vi "main.vi"() -> ()   [LabVIEW 2021]
uses:
  data_cluster_typedef.ctl
  states_enum_typedef.ctl
  <vilib>/Utility/file.llb/Write Delimited Spreadsheet (DBL).vi
  <vilib>/Instr/_visa.llb/VISA Configure Serial Port (Instr).vi
  <vilib>/Utility/file.llb/Read Delimited Spreadsheet (DBL).vi
panel:
  out "XY Graph":cluster{"Time":dbl[], "Displacement":dbl[]}(graph)
  out "Connected?":bool
  in  "Serial Port":refnum<visa-resource-name>
  in  "Disconnect":bool
  in  "Connect":bool
  in  "Clear":bool
  in  "Save":bool
  in  "Load":bool
  in  "Exit":bool
  # "Creep Deformation"
  # "1) Connect your creep machine to the computer\n2) Select the appropriate serial port from the list\n3) Click \"Connect\"\n4) Run your experiment\n5) Save the data if desired, then clear the chart\n6) When all experiments are done, click \"Disconnect\""
  # "V1.1"
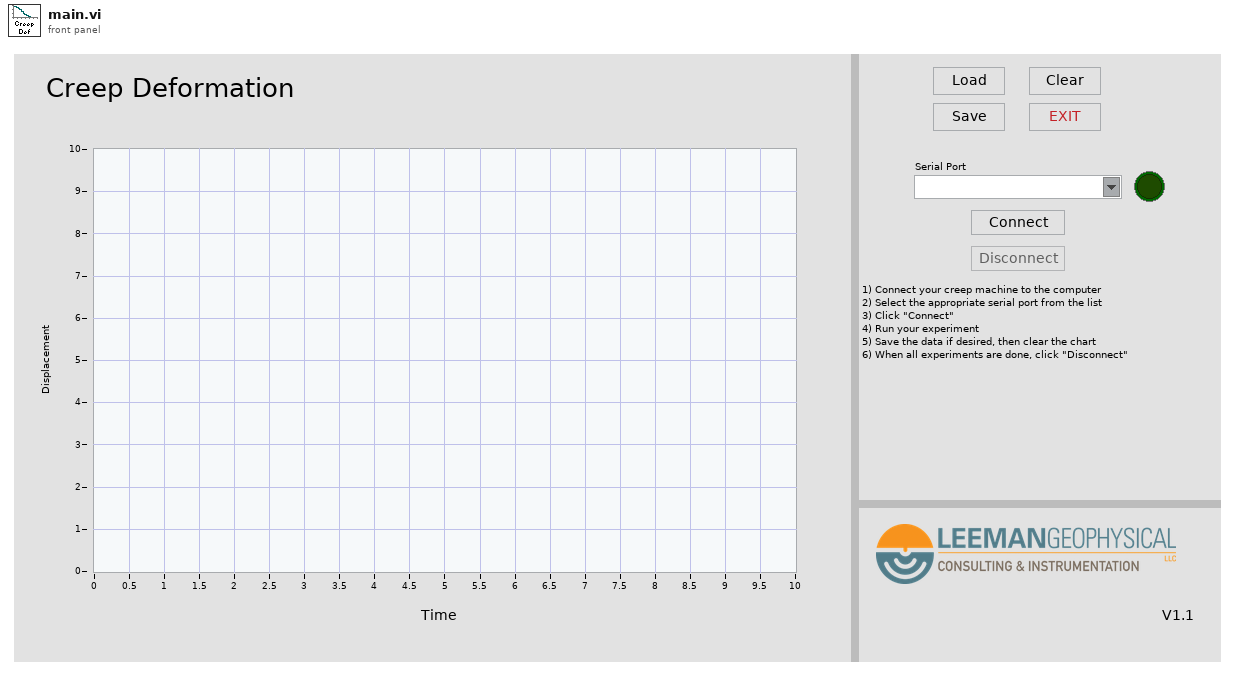
[diagram p1: front panel]
types:
  T1 = enum8{"Enabled", "Disabled", "Disabled and Grayed Out"}
  T2 = typedef "states_enum_typedef.ctl" = enum16{"Shutdown", "Update", "Initialize", "Clear", "Save", "Connect", "Disconnect", "Load", "Wait"}
  T3 = typedef "data_cluster_typedef.ctl" = cluster{"Time":dbl[], "Displacement":dbl[]}
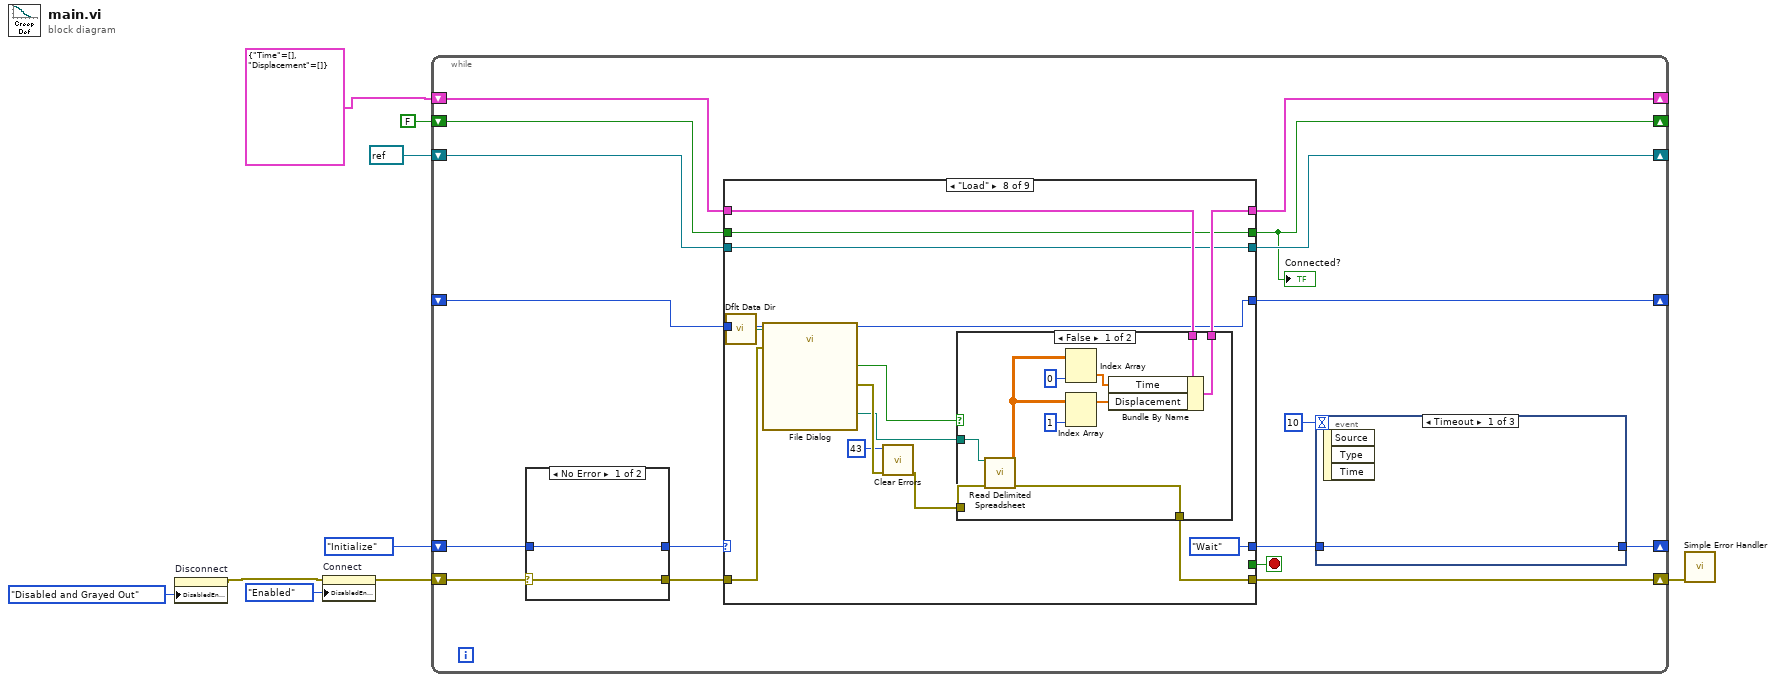
[diagram p0: block diagram]
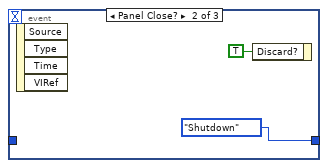
[diagram p2: hidden frame]
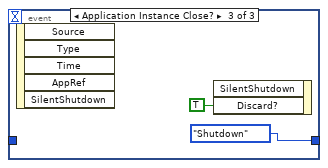
[diagram p3: hidden frame]
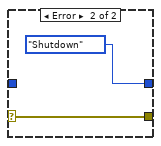
[diagram p4: hidden frame]
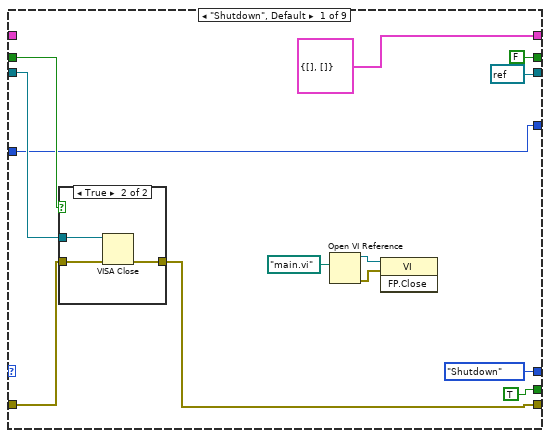
[diagram p5: hidden frame]
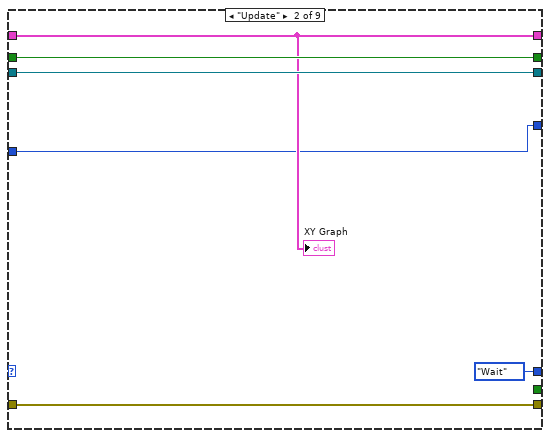
[diagram p7: hidden frame]
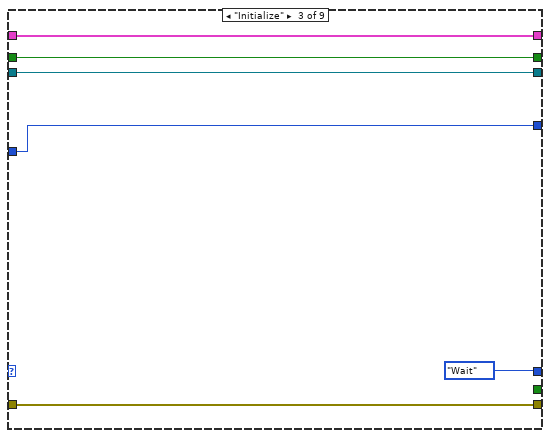
[diagram p8: hidden frame]
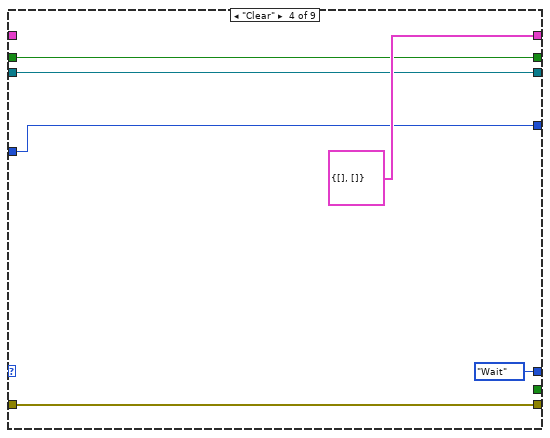
[diagram p9: hidden frame]
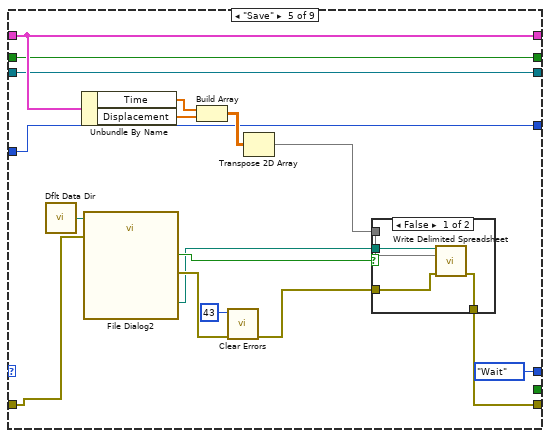
[diagram p10: hidden frame]
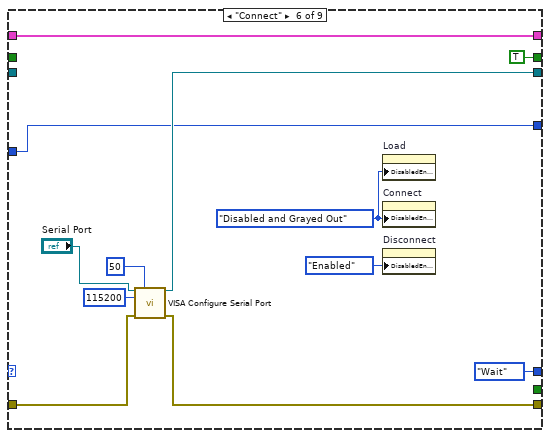
[diagram p12: hidden frame]
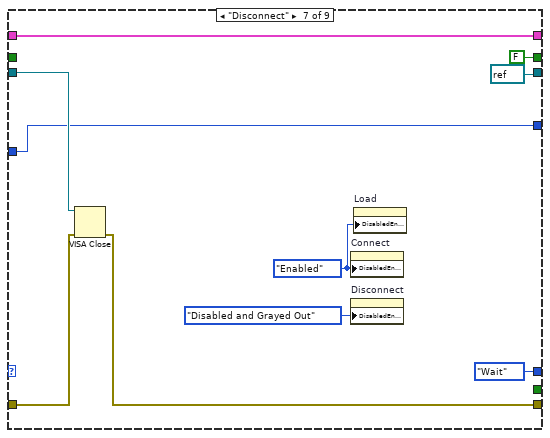
[diagram p13: hidden frame]
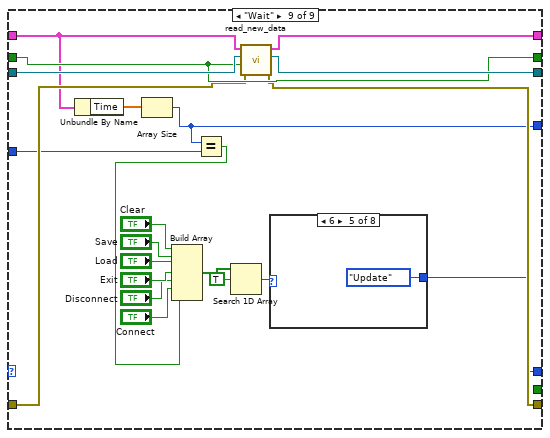
[diagram p15: hidden frame]
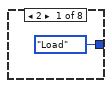
[diagram p16: hidden frame]
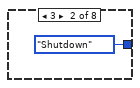
[diagram p17: hidden frame]
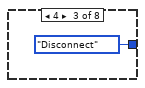
[diagram p18: hidden frame]
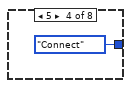
[diagram p19: hidden frame]
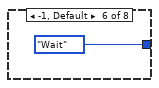
[diagram p20: hidden frame]
diagram:
  n1 = property on="Disconnect" class="Bool"("DisabledEnum"=T1."Disabled and Grayed Out" ("Disabled")) -> (error out=w2:errorcluster)  [unwired: 2 in, 1 out]
  n2 = property on="Connect" class="Bool"(error in=w2, "DisabledEnum"=T1."Enabled" ("Disabled")) -> (error out=w1:errorcluster)  [unwired: 1 in, 1 out]
  n3 = while {
    shift-right: [w11] -> _
    shift-left: states_enum_typedef."Initialize" -> [w25]
    shift-right: [w17] -> w5
    shift-left: w1 -> [w26]
    shift-right: [w19] -> _
    shift-left: T3 {"Time"=[], "Displacement"=[]} -> [w22]
    shift-right: [w16] -> _
    shift-left: FALSE -> [w21]
    shift-right: [w18] -> _
    shift-left: refnum<visa-resource-name> refnum ("Serial Port") -> [w20]
    shift-right: [w14] -> _
    shift-left: _ -> [w13]
    stop <- w15 stop-if-true
    n4 = case shown="No Error" w26 {
      selector: w26 -> [w32 w34]
      tunnel: w25 -> [w33 _]
      tunnel: [w33 states_enum_typedef."Shutdown"] -> w24
      tunnel: [w32 w34] -> w23
      frame No Error {
      }
      frame Error {
      }
    }
    n5 = case shown="\"Load\"" w24 {
      tunnel: w23 -> [w46 w55 w61 w66 w74 w101 w113 w118 w148]
      tunnel: w22 -> [_ w54 w64 _ w81 w98 w110 w128 w145]
      tunnel: w21 -> [w48 w58 w63 w69 w80 _ _ w126 w149]
      tunnel: w20 -> [w47 w57 w62 w68 w79 _ w114 w125 w150]
      tunnel: [T3 {"Time"=[], "Displacement"=[]} ("Data Cluster Out") w54 w64 T3 {"Time"=[], "Displacement"=[]} w81 w98 w110 w127 w152] -> w19
      tunnel: [FALSE w58 w63 w69 w80 TRUE FALSE w126 w149] -> w16
      tunnel: [refnum<visa-resource-name> refnum ("VISA out") w57 w62 w68 w79 w99 refnum<visa-resource-name> refnum ("VISA resource name out") w125 w151] -> w18
      tunnel: [w40 w55 w61 w66 w83 w100 w112 w124 w147] -> w17
      tunnel: [states_enum_typedef."Shutdown" states_enum_typedef."Wait" states_enum_typedef."Wait" states_enum_typedef."Wait" states_enum_typedef."Wait" states_enum_typedef."Wait" states_enum_typedef."Wait" states_enum_typedef."Wait" w146] -> w10
      tunnel: [TRUE _ _ _ _ _ _ _ _] -> w15
      tunnel: [w36 w53 w59 w65 w78 w94 w106 w122 w143] -> w14
      tunnel: w13 -> [w36 w53 w59 w65 w78 w94 w106 w122 w142]
      frame "Shutdown", Default {
        n6 = case shown="True" w48 {
          tunnel: w47 -> [_ w52]
          tunnel: w46 -> [w49 w51]
          tunnel: [w49 w50] -> w40
          frame False {
          }
          frame True {
            n7 = VISA Close(VISA resource name=w52, error in (no error)=w51) -> (error out=w50:errorcluster)
          }
        }
        n8 = Open VI Reference(vi path=path "main.vi") -> (vi reference=w38:refnum<vi>, error out=w37:errorcluster)  [unwired: 5 in]
        n9 = invoke class="VI" method="FP.Close"(reference=w38, error in=w37) -> ()  [unwired: 1 in, 3 out]
      }
      frame "Update" {
        "XY Graph" <- w54
      }
      frame "Initialize" {
      }
      frame "Clear" {
      }
      frame "Save" {
        n10 = call <vilib>:"Dflt Data Dir.vi"() -> ("App:Default Data Directory"=w77:path)
        n11 = Unbundle By Name(w81) -> ("Time"=w87:dbl[], "Displacement"=w86:dbl[])
        n12 = call "File Dialog2"("start path"=w77, "error in"=w74) -> ("selected path"=w71:path, "cancelled"=w73:bool, "error out"=w76:errorcluster)  [unwired: 10 in, 1 out]
        n13 = Build Array(w87, w86) -> (w85:dbl[][])
        n14 = call <vilib>:"Clear Errors.vi"("error in (no error)"=w76, "specific error code to clear (0: all)"=43) -> ("error out"=w72:errorcluster)  [unwired: 4 in, 1 out]
        n15 = Transpose 2D Array(2D array=w85) -> (transposed array=w84:dbl[][])
        n16 = case shown="False" w73 {
          tunnel: w84 -> [w91 _]
          tunnel: [w90 w92] -> w83
          tunnel: w72 -> [w89 w92]
          tunnel: w71 -> [w88 _]
          frame False {
            n17 = call-poly <vilib>:"Write Delimited Spreadsheet.vi"("file path (dialog if empty)"=w88, "2D data"=w91, "error in (no error)"=w89) -> ("error out"=w90:errorcluster)  [unwired: 11 in, 1 out]
          }
          frame True {
          }
        }
      }
      frame "Connect" {
        w93 = T1."Disabled and Grayed Out" ("Disabled")
        n18 = call-poly "VISA Configure Serial Port"("VISA resource name"="Serial Port", "timeout (10sec)"=u32 50, "baud rate (9600)"=u32 115200, "error in (no error)"=w101) -> ("VISA resource name out"=w99:refnum<visa-resource-name>, "error out"=w100:errorcluster)  [unwired: 10 in]
        n19 = property on="Load" class="Bool"("DisabledEnum"=w93) -> ()  [unwired: 2 in, 2 out]
        n20 = property on="Connect" class="Bool"("DisabledEnum"=w93) -> ()  [unwired: 2 in, 2 out]
        n21 = property on="Disconnect" class="Bool"("DisabledEnum"=T1."Enabled" ("Disabled")) -> ()  [unwired: 2 in, 2 out]
      }
      frame "Disconnect" {
        w105 = T1."Enabled" ("Disabled")
        n22 = VISA Close(VISA resource name=w114, error in (no error)=w113) -> (error out=w112:errorcluster)
        n23 = property on="Connect" class="Bool"("DisabledEnum"=w105) -> ()  [unwired: 2 in, 2 out]
        n24 = property on="Disconnect" class="Bool"("DisabledEnum"=T1."Disabled and Grayed Out" ("Disabled")) -> ()  [unwired: 2 in, 2 out]
        n25 = property on="Load" class="Bool"("DisabledEnum"=w105) -> ()  [unwired: 2 in, 2 out]
      }
      frame "Load" {
        n26 = call <vilib>:"Dflt Data Dir.vi"() -> ("App:Default Data Directory"=w120:path)
        n27 = call "File Dialog"("start path"=w120, "error in"=w118) -> ("selected path"=w115:path, "cancelled"=w116:bool, "error out"=w121:errorcluster)  [unwired: 10 in, 1 out]
        n28 = call <vilib>:"Clear Errors.vi"("error in (no error)"=w121, "specific error code to clear (0: all)"=43) -> ("error out"=w117:errorcluster)  [unwired: 4 in, 1 out]
        n29 = case shown="False" w116 {
          tunnel: w128 -> [w133 w140]
          tunnel: [w132 w140] -> w127
          tunnel: w117 -> [w131 w139]
          tunnel: [w130 w139] -> w124
          tunnel: w115 -> [w129 _]
          frame False {
            n30 = call-poly <vilib>:"Read Delimited Spreadsheet.vi"("file path (dialog if empty)"=w129, "error in (no error)"=w131) -> ("all rows"=w136:dbl[][], "error out"=w130:errorcluster)  [unwired: 8 in, 4 out]
            n31 = Index Array(array=w136, index (col)=0 ("disabled index (col)")) -> (element=w135:dbl[])  [unwired: 1 in]
            n32 = Index Array(array=w136, index (col)=1 ("disabled index (col)")) -> (element=w134:dbl[])  [unwired: 1 in]
            n33 = Bundle By Name(cluster=w133, "Time"=w135, "Displacement"=w134) -> (w132:T3)
          }
          frame True {
          }
        }
      }
      frame "Wait" {
        n34 = Unbundle By Name(w145) -> ("Time"=w144:dbl[])
        n35 = Array Size(array=w144) -> (size(s)=w143:i32)
        n36 = Equal?(x=w143, y=w142) -> (x = y?=w141:bool)
        n37 = Build Array("Clear", "Save", "Load", "Exit", "Disconnect", "Connect", w141) -> (w155:bool[])
        n38 = Search 1D Array(1D array=w155, element=TRUE) -> (index of element=w153:i32)  [unwired: 1 in]
        n39 = call "read_new_data.vi"("Error In"=w148, "connected?"=w149, "VISA in"=w150, "Data Cluster In"=w145) -> ("error out"=w147:errorcluster, "VISA out"=w151:refnum<visa-resource-name>, "Data Cluster Out"=w152:T3)  [unwired: 5 in]
        n40 = case shown="6" w153 {
          tunnel: [states_enum_typedef."Load" states_enum_typedef."Shutdown" states_enum_typedef."Disconnect" states_enum_typedef."Connect" states_enum_typedef."Update" states_enum_typedef."Wait" states_enum_typedef."Clear" states_enum_typedef."Save"] -> w146
          frame 2 {
          }
          frame 3 {
          }
          frame 4 {
          }
          frame 5 {
          }
          frame 6 {
          }
          frame -1, Default {
          }
          frame 0 {
          }
          frame 1 {
          }
        }
      }
    }
    "Connected?" <- w16
    n41 = event shown="[0] Timeout" {
      selector: _ -> [_ _ _]
      dyn-events: _ -> [_ _ _]
      timeout: 10 -> [_ _ _]
      tunnel: [w27 states_enum_typedef."Shutdown" states_enum_typedef."Shutdown"] -> w11
      tunnel: w10 -> [w27 _ _]
      event Timeout {
        n42 = event-data() -> ()  [unwired: 1 in, 3 out]
      }
      event Panel Close? {
        n43 = event-data() -> ()  [unwired: 1 in, 4 out]
        n44 = event-data("Discard?"=TRUE) -> ()  [unwired: 1 in, 1 out]
      }
      event Application Instance Close? {
        n45 = event-data() -> ()  [unwired: 1 in, 5 out]
        n46 = event-data("Discard?"=TRUE) -> ()  [unwired: 2 in, 1 out]
      }
    }
  }
  n47 = call <vilib>:"Simple Error Handler.vi"("error in (no error)"=w5) -> ()  [unwired: 4 in, 5 out]
